vi "LaunchATE.vi"   [LabVIEW 2019]
uses:
  Components/ViPER.lvlibp/1abvi3w/ProjectTemplates/Source/Core/ViPER/Components_Src/ViPER/ViPER.lvclass
panel:
  # "Test Executive"
types:
  T1 = enum32{"Invalid", "Standard", "Closed", "Hidden", "Minimized", "Maximized"}
  T2 = enum32{"invalid app kind", "Development System", "Run Time System", "Student Edition", "Embedded LabVIEW", "Evaluation", "Custom"}
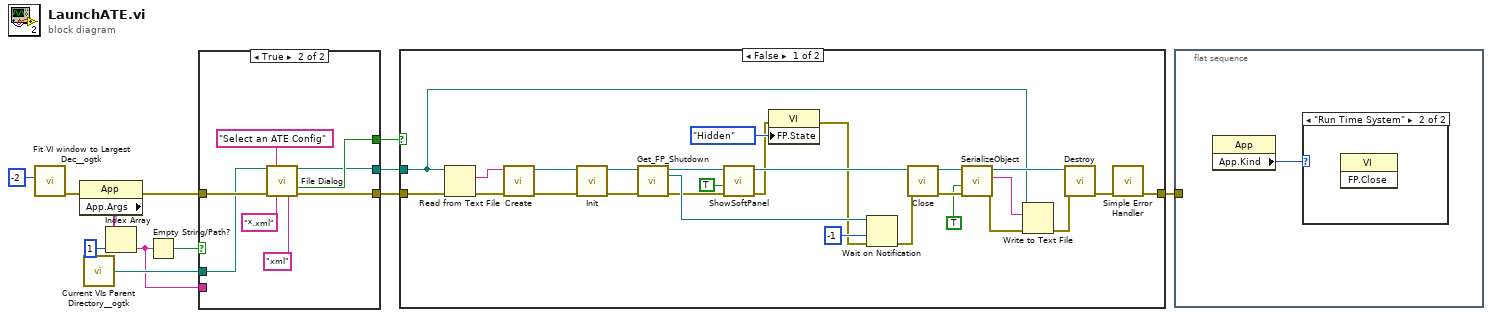
[diagram p0: block diagram]
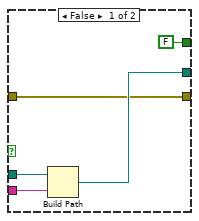
[diagram p2: hidden frame]
diagram:
  n1 = call <userlib>:"Fit VI window to Largest Dec__ogtk.vi"("border spacing (2 px)"=-2) -> ("error out"=w8:errorcluster)  [unwired: 5 in, 1 out]
  n2 = property class="App"(error in=w8) -> (error out=w3:errorcluster, "App.Args"=w10:string[])  [unwired: 1 in, 1 out]
  n3 = call <userlib>:"Current VIs Parent Directory__ogtk.vi"() -> ("Parent Directory (+ Relative)"=w6:path)  [unwired: 5 in]
  n4 = Index Array(array=w10, index=1) -> (element=w5:string)
  n5 = Empty String/Path?(string/path=w5) -> (empty?=w7:bool)
  n6 = case shown="True" w7 {
    tunnel: w6 -> [w17 w23]
    tunnel: w5 -> [w16 _]
    tunnel: [w15 w19] -> w4
    tunnel: w3 -> [w13 w25]
    tunnel: [w13 w24] -> w2
    tunnel: [FALSE ("cancelled") w20] -> w1
    frame False {
      n7 = Build Path(base path=w17, name or relative path=w16) -> (appended path=w15:path)
    }
    frame True {
      n8 = call "File Dialog"("start path"=w23, "prompt"="Select an ATE Config", "error in"=w25, "pattern (all files)"="*.xml", "pattern label"="xml") -> ("selected path"=w19:path, "cancelled"=w20:bool, "error out"=w24:errorcluster)  [unwired: 7 in, 1 out]
    }
  }
  n9 = case shown="False" w1 {
    tunnel: [w40 w53] -> w12
    tunnel: w2 -> [w36 w53]
    tunnel: w4 -> [w27 _]
    frame False {
      n10 = Read from Text File(file (use dialog)=w27, error in=w36) -> (text=w34:string, error out=w35:errorcluster)  [unwired: 2 in, 2 out]
      n11 = call "Create.vi"("error in (no error)"=w35, "Config XML"=w34) -> ("error out"=w49:errorcluster, "reference out"=w50:refnum<class "ViPER.lvclass">)  [unwired: 8 in]
      n12 = call-dynamic "Init.vi"("error in (no error)"=w49, "reference in"=w50) -> ("error out"=w47:errorcluster, "reference out"=w48:refnum<class "ViPER.lvclass">)  [unwired: 8 in]
      n13 = call "Get_FP_Shutdown.vi"("ViPER_Base in"=w48, "error in (no error)"=w47) -> ("ViPER_Base out"=w45:refnum<class "ViPER.lvclass">, "SoftFP_Shutdown"=w46:refnum<notifier>, "error out"=w44:errorcluster)  [unwired: 9 in, 2 out]
      n14 = call-dynamic "ShowSoftPanel.vi"("error in (no error)"=w44, "Floating"=TRUE, "Driver in"=w45) -> ("error out"=w38:errorcluster, "Driver out"=w43:refnum<class "ViPER.lvclass">)  [unwired: 6 in, 1 out]
      n15 = property class="VI"(error in=w38, "FP.State"=T1."Hidden" ("Front Panel Window:State")) -> (error out=w37:errorcluster)  [unwired: 1 in, 1 out]
      n16 = Wait on Notification(notifier=w46, timeout in ms (-1)=-1, error in (no error)=w37) -> (error out=w52:errorcluster)  [unwired: 1 in, 3 out]
      n17 = call-dynamic "Close.vi"("error in (no error)"=w52, "reference in"=w43) -> ("error out"=w33:errorcluster, "reference out"=w32:refnum<class "ViPER.lvclass">)  [unwired: 8 in]
      n18 = call-dynamic "SerializeObject.vi"("error in (no error)"=w33, "Pretty Print?"=TRUE, "ViPER_Base in"=w32) -> ("error out"=w30:errorcluster, "Object XML"=w28:string, "ViPER_Base out"=w31:refnum<class "ViPER.lvclass">)  [unwired: 6 in]
      n19 = Write to Text File(file (use dialog)=w27, text=w28, error in=w30) -> (error out=w29:errorcluster)  [unwired: 1 in, 2 out]
      n20 = call "Destroy.vi"("error in (no error)"=w29, "reference in"=w31) -> ("error out"=w42:errorcluster)  [unwired: 9 in]
      n21 = call <vilib>:"Simple Error Handler.vi"("error in (no error)"=w42) -> ("error out"=w40:errorcluster)  [unwired: 4 in, 4 out]
    }
    frame True {
    }
  }
  n22 = flat-sequence {
    tunnel: w12 -> [_]
    frame #0 {
      n23 = property class="App"() -> ("App.Kind"=w54:T2)  [unwired: 2 in, 2 out]
      n24 = case shown="\"Run Time System\"" w54 {
        frame "invalid app kind", Default {
        }
        frame "Run Time System" {
          n25 = invoke class="VI" method="FP.Close"() -> ()  [unwired: 3 in, 3 out]
        }
      }
    }
  }
